vi "PC Code_testtransmit.vi"() -> ()   [LabVIEW 2014]
uses:
  <vilib>/Instr/_visa.llb/VISA Flush IO Buffer Mask.ctl
panel:
  out "Running?":bool
  in  "Input String 2":string="Hello"
  out "Input Indicator":string
  in  "Input String":string="World"
  in  "stop":bool caption="ESTOP"
  out "String Received":string
  in  "VISA resource name":refnum<visa-resource-name>="COM6"
  in  "error in":errorcluster
  out "Battery\nVolts":i16
  out "Mode":i16=1
  out "Local\nHeading":i16=90
  out "Desired \nVelocity":i16=5
  out "Dist":i16
  out "IR Index":i32
  out "error out":errorcluster
  out "return count":u32
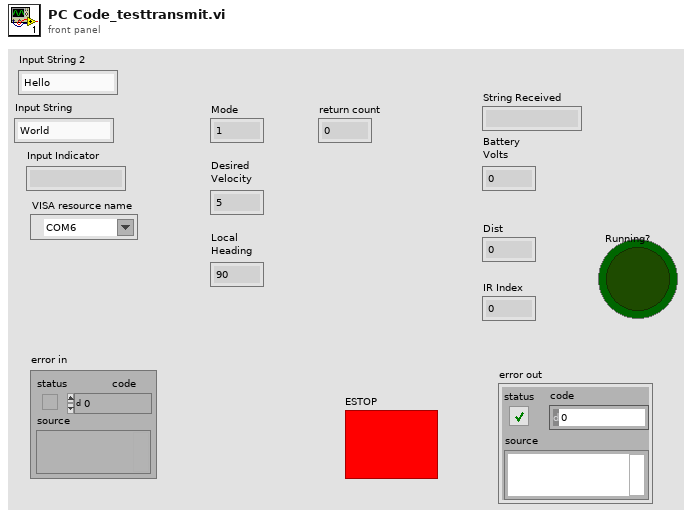
[diagram p1: front panel]
types:
  T1 = typedef "VISA Flush IO Buffer Mask.ctl" = u16
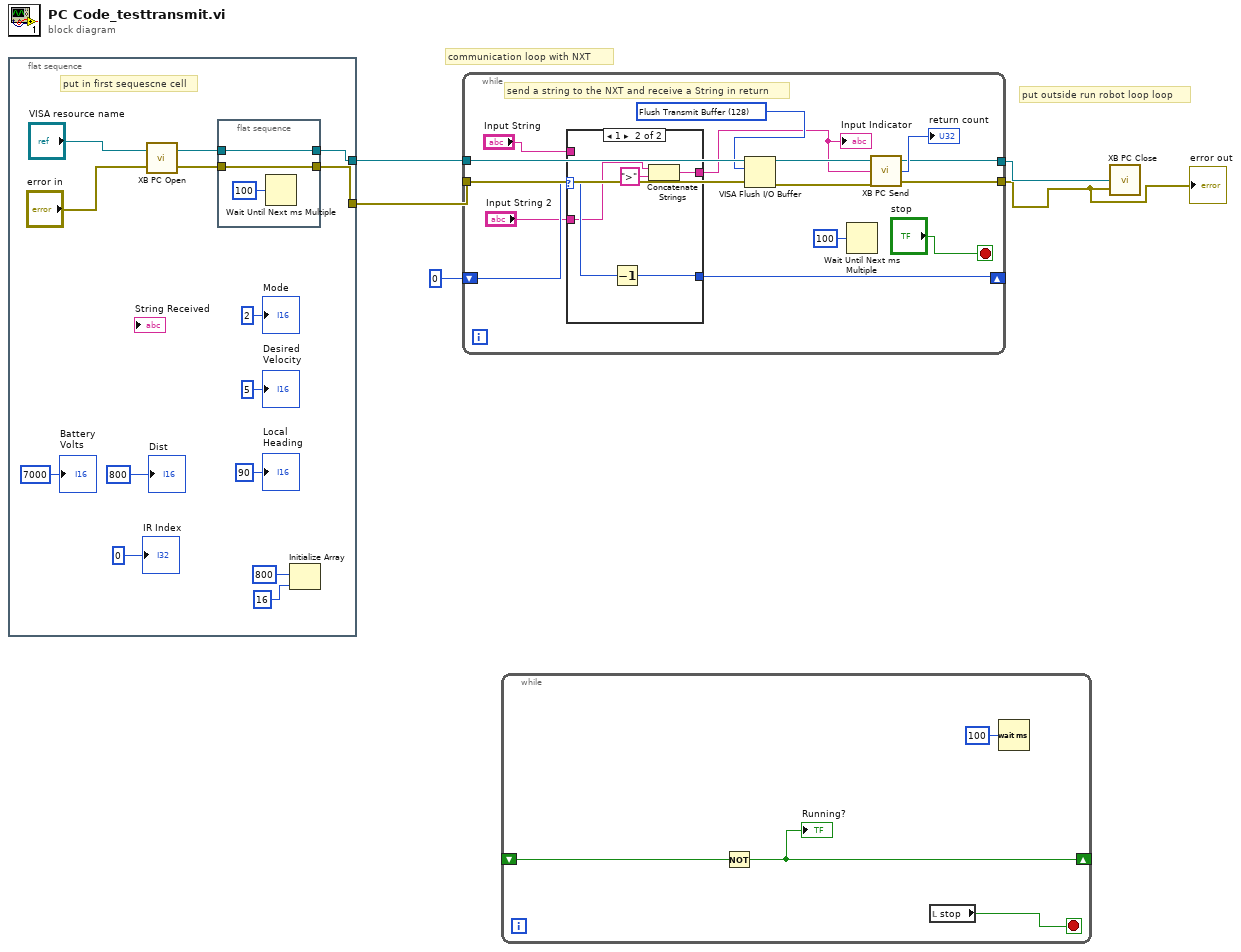
[diagram p0: block diagram]
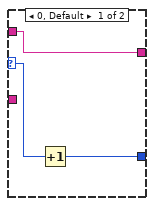
[diagram p2: hidden frame]
diagram:
  # "put outside run robot loop loop"
  # "communication loop with NXT"
  n1 = flat-sequence {
    tunnel: [w7] -> w3
    tunnel: [w6] -> w2
    frame #0 {
      # "put in first sequescne cell"
      n2 = call "XB PC Open.vi"("error in (no error)"="error in", "VISA resource name"="VISA resource name") -> ("error out"=w18:errorcluster, "VISA resource name out"=w19:refnum<visa-resource-name>)
      n3 = flat-sequence {
        tunnel: w19 -> [w20]
        tunnel: w18 -> [w21]
        tunnel: [w21] -> w7
        tunnel: [w20] -> w6
        frame #0 {
          n4 = Wait Until Next ms Multiple(millisecond multiple=u32 100) -> ()  [unwired: 1 out]
        }
      }
      n5 = Initialize Array(i16 800, 16 ("dimension size")) -> ()  [unwired: 1 out]
      "Battery\nVolts" <- i16 7000 ("Battery\nVolts")
      "Mode" <- i16 2 ("Mode")
      "Local\nHeading" <- i16 90 ("Local\nHeading")
      "Desired \nVelocity" <- i16 5 ("Desired \nVelocity")
      "Dist" <- i16 800 ("Dist")
      "IR Index" <- 0 ("IR Index")
    }
  }
  n6 = while {
    tunnel: w2 -> [w32]
    tunnel: w3 -> [w30]
    tunnel: [w33] -> w4
    tunnel: [w34] -> w5
    shift-right: [w26] -> _
    shift-left: 0 -> [w27]
    stop <- "stop" stop-if-true
    w28 = T1 128 items=["Flush Receive Buffer"=16, "Write Transmit Buffer to Device"=32, "Flush Receive Buffer (No I/O)"=64, "Flush Transmit Buffer"=128] ("Mask")
    # "send a string to the NXT and receive a String in return"
    n7 = case shown="1" w27 {
      selector: w27 -> [w40 w44]
      tunnel: [w39 w45] -> w26
      tunnel: "Input String 2" -> [_ w42]
      tunnel: "Input String" -> [w38 _]
      tunnel: [w38 w41] -> w23
      frame 0, Default {
        n8 = Increment(x=w40) -> (x+1=w39:i32)
      }
      frame 1 {
        n9 = Decrement(x=w44) -> (x-1=w45:i32)
        n10 = Concatenate Strings(w42, ">" ("string")) -> (w41:string)
      }
    }
    "Input Indicator" <- w23
    n11 = VISA Flush I/O Buffer(VISA resource name=w32, mask (16)=w28, error in (no error)=w30) -> (VISA resource name out=w31:refnum<visa-resource-name>, error out=w29:errorcluster)
    n12 = Wait Until Next ms Multiple(millisecond multiple=u32 100) -> ()  [unwired: 1 out]
    n13 = call "XB PC Send.vi"("error in (no error)"=w29, "String"=w23, "VISA resource name"=w31) -> ("error out"=w33:errorcluster, "return count"=→"return count":u32, "VISA resource name out"=w34:refnum<visa-resource-name>)
  }
  "error out" <- w4
  n14 = while {
    shift-right: [w48] -> _
    shift-left: _ -> [w49]
    stop <- w46 stop-if-true
    n15 = Not(x=w49) -> (.not. x?=w48:bool)
    "Running?" <- w48
    n16 = local read "stop"() -> (w46:bool)
    n17 = Wait (ms)(milliseconds to wait=u32 100) -> ()  [unwired: 1 out]
  }
  n18 = call "XB PC Close.vi"("error in (no error)"=w4, "VISA resource name"=w5) -> ()
